vi "Robot Global Data.vi"() -> ()   [LabVIEW 2018]
doc: "This global VI can contain as many global variables as you need. Place a control on the panel, give it a good name. To read or write to it from a VI, drag the icon to the diagram of that VI. You can also drag from the project. Click on the node to change which global you access. You shouldn't have multiple locations writing to a global or it will cause a race-condition."
uses:
  <vilib>/Rock Robotics/WPI/Camera/WPI_CameraImageSize.ctl
  <vilib>/Rock Robotics/WPI/DriverStation/WPI_DriverStationRobotMode2.ctl
  Which Robot Enum.ctl
panel:
  out "Back HAB 3 Limit Switch":bool
  out "Front HAB 3 Limit Switch":bool
  out "HAB Module Actual Velocity":dbl
  out "HAB Back Cylinders Extended?":bool
  out "HAB Front Cylinders Extended?":bool
  out "HAB Bk Spd Encoder Start Value":dbl
  out "Roll (forward/backward tipping)":dbl
  out "Pitch (left/right tipping)":dbl
  out "Right Encoder in Inches":dbl
  out "Left Encoder in Inches":dbl
  out "Right Encoder Val. Initial":dbl
  out "Left Encoder Val. Initial":dbl
  out "Kick Hatch in Auto":bool
  in  "Which Robot?":T1
  out "Cancel the Motion Profile?":bool
  out "Run the Motion Profile?":bool=TRUE
  out "Right Train MP Status":T2
  out "Left Train MP Status":T2
  out "Right Encoder in Enc. Vals":dbl
  out "Left Encoder in Enc. Vals":dbl
  out "Yaw (clockwise/counter-clockwise)":dbl
  out "Hatch Encoder Start Value":dbl
  in  "Hatch Motor Encoder":dbl
  out "Driver VS Vision Control":bool
  out "Right Drive Joystick Y":dbl
  out "Right Drive Joystick X":dbl
  out "Left Drive Joystick Y":dbl
  out "Left Drive Joystick X":dbl
  in  "Robot Mode":T3
  in  "image size":T4=enum."320x240"
  in  "Enable Vision":bool
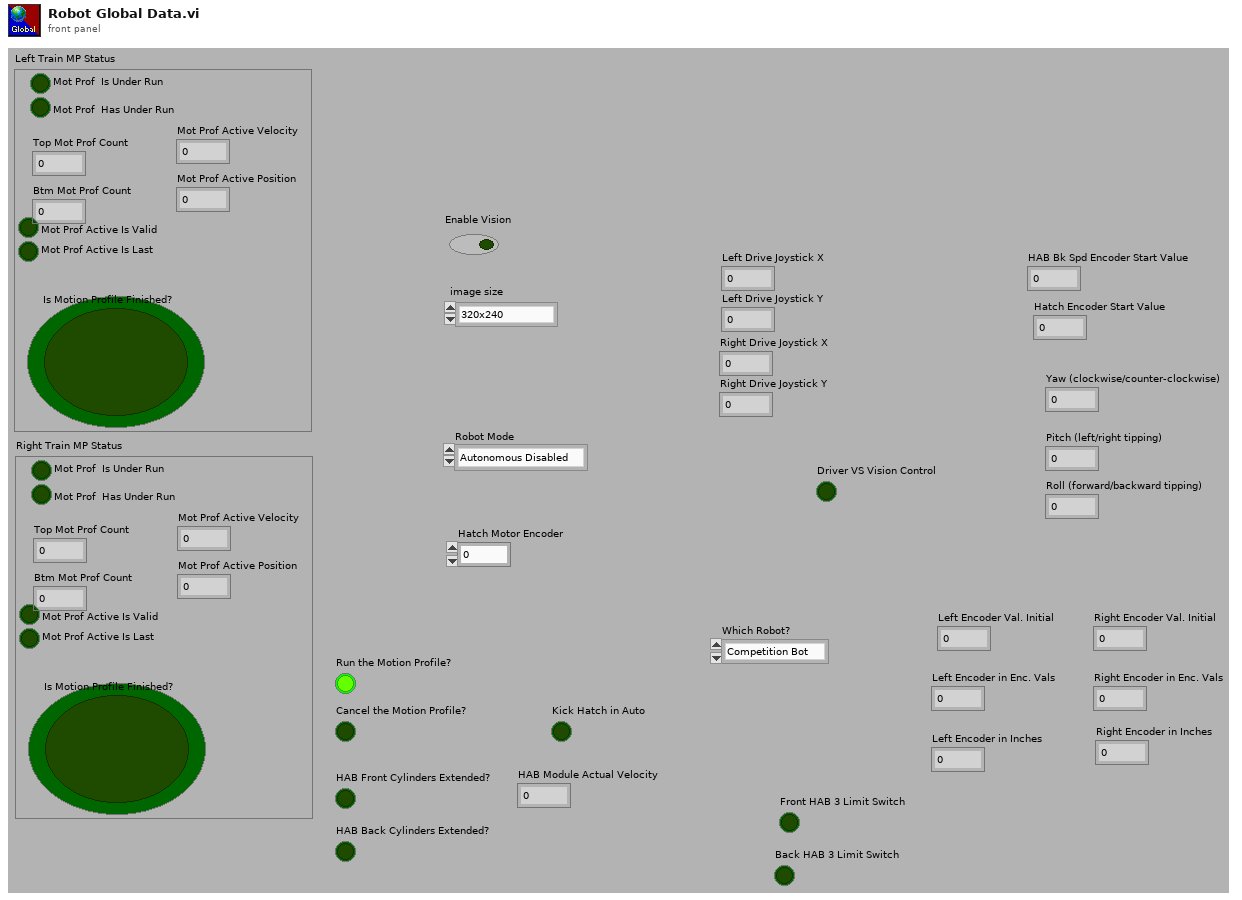
[diagram p1: front panel]
types:
  T1 = typedef "Which Robot Enum.ctl" = enum16{"Competition Bot", "Practice Bot", "Code Bot"}
  T2 = cluster{"Mot Prof Active Velocity":dbl, "Mot Prof Active Position":dbl, "Mot Prof  Is Under Run":bool, "Mot Prof  Has Under Run":bool, "Mot Prof Active Is Last":bool, "Mot Prof Active Is Valid":bool, "Top Mot Prof Count":i32, "Btm Mot Prof Count":i32, "Is Motion Profile Finished?":bool}
  T3 = typedef "WPI_DriverStationRobotMode2.ctl" = enum16{"Autonomous Disabled", "Autonomous Enabled", "Teleop Disabled", "Teleop Enabled", "Disconnected", "Finish", "Test Disabled", "Test Enabled", "Emergency Stopped"}
  T4 = typedef "WPI_CameraImageSize.ctl" = enum16{"640x480", "320x240", "160x120", "Custom"}
diagram:
